vi "Sklej Wfm.vi"(6 "zerowy?":bool, 8 "error in (no error)":errorcluster, 9 "Wfm Bufor in":waveform(dbl)[](array[waveform]), 10 "New data":waveform(dbl)[](array[waveform])) -> (0 "error out":errorcluster, 1 "Wfm Bufor out":waveform(dbl)[](array[waveform]))   [LabVIEW 2014]
doc: "Skleja wektory Waveform do bufora Wfm"
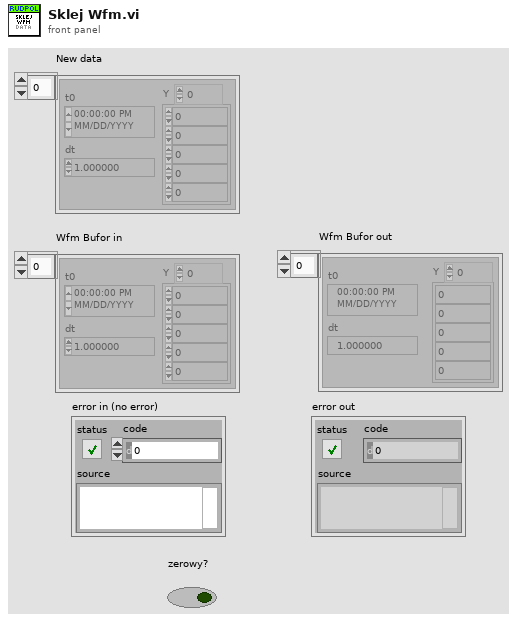
[diagram p1: front panel]
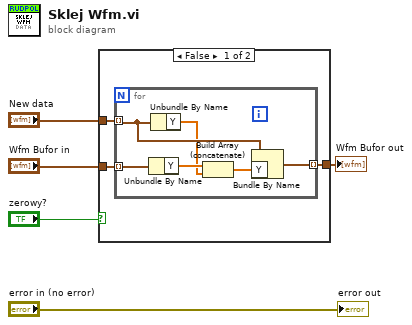
[diagram p0: block diagram]
diagram:
  n1 = case shown="False" "zerowy?" {
    tunnel: [w6 w15] -> w5
    tunnel: "New data" -> [w8 w15]
    tunnel: "Wfm Bufor in" -> [w7 _]
    frame False {
      n2 = for {
        tunnel: w7 -> [w14] mode=indexing
        tunnel: w8 -> [w12] mode=indexing
        tunnel: [w13] -> w6 mode=indexing
        n3 = Unbundle By Name(w14) -> ("Y"=w11:dbl[])
        n4 = Unbundle By Name(w12) -> ("Y"=w10:dbl[])
        n5 = Build Array (concatenate)(w11, w10) -> (w9:dbl[])
        n6 = Bundle By Name(cluster=w12, "Y"=w9) -> (w13:waveform(dbl))
      }
    }
    frame True {
    }
  }
  "Wfm Bufor out" <- w5
  "error out" <- "error in (no error)"
